vi "Read Stream standard output.vi"(6 "Timout (s)":i32, 8 "error in (no error)":errorcluster, 9 "Output ref":refnum<vi>, 10 "reader":refnum<k24>, 11 "stream":refnum<k24>) -> (0 "error out":errorcluster)   [LabVIEW 2016, in "labssh_thijs.lvlib" / "LabSSH.lvlib"]
uses:
  LabSSH.lvlib
  C:/Users/thosman/Documents/Development/Labview/ssh in labview/LabSSH/LabSSH/References/Renci.SshNet.dll
  LabSSH/LabSSH/References/Renci.SshNet.dll
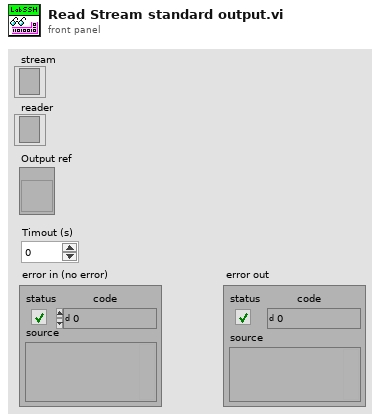
[diagram p1: front panel]
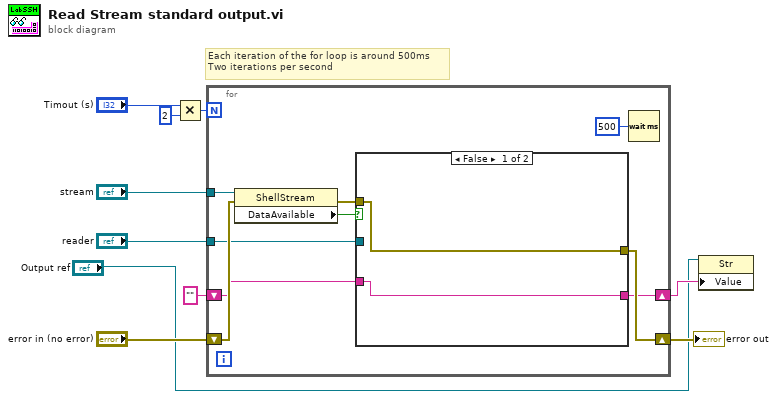
[diagram p0: block diagram]
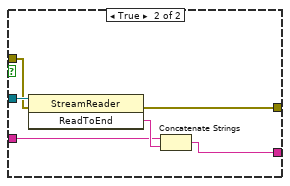
[diagram p2: hidden frame]
diagram:
  # "Each iteration of the for loop is around 500ms\nTwo iterations per second"
  n1 = Multiply(x="Timout (s)", y=2) -> (x*y=w9:i32)
  n2 = for {
    N: w9 -> [_]
    tunnel: "stream" -> [w18]
    tunnel: "reader" -> [w15]
    shift-right: [w13] -> w4
    shift-left: "error in (no error)" -> [w16]
    shift-right: [w11] -> w3
    shift-left: "" -> [w12]
    n3 = property class="ShellStream"(reference=w18, error in=w16) -> (error out=w14:errorcluster, "DataAvailable"=w17:bool)  [unwired: 1 out]
    n4 = case shown="False" w17 {
      tunnel: w15 -> [_ w27]
      tunnel: w14 -> [w21 w26]
      tunnel: [w21 w25] -> w13
      tunnel: w12 -> [w20 w22]
      tunnel: [w20 w23] -> w11
      frame False {
      }
      frame True {
        n5 = invoke class="StreamReader" method="ReadToEnd"(reference=w27, error in=w26) -> (error out=w25:errorcluster, "ReadToEnd"=w24:string)  [unwired: 1 in, 1 out]
        n6 = Concatenate Strings(w22, w24) -> (w23:string)
      }
    }
    n7 = Wait (ms)(milliseconds to wait=u32 500) -> ()  [unwired: 1 out]
  }
  "error out" <- w4
  n8 = property class="Str"(reference="Output ref", "Value"=w3) -> ()  [unwired: 1 in, 2 out]
